vi "Launcher Nested Actor Caller.vi"(8 "error in (no error)":errorcluster, 10 "Sidebar":refnum<vi>, 11 "Post Analysis in":refnum<class "Post Analysis.lvclass">) -> (0 "error out":errorcluster, 3 "Post Analysis out":refnum<class "Post Analysis.lvclass">)   [LabVIEW 2023, in "Data Analysis.lvlib" / "Post Analysis.lvlib" / "Post Analysis.lvclass"]
uses:
  Post Analysis.lvclass
  Post Analysis.lvclass/Post Analysis.ctl
  <vilib>/ActorFramework/Message Enqueuer/Message Enqueuer.lvclass/Message Enqueuer.ctl
  Test Info/Test Info/Test Info.lvclass
  Test Info/Test Info/Test Info.lvclass/Test Info.ctl
  Error Log/Error Log/Error Log.lvclass
  Error Log/Error Log/Error Log.lvclass/Error Log.ctl
  FE FF Frame/FE FF Frame/FE FF Frame.lvclass
  FE FF Frame/FE FF Frame/FE FF Frame.lvclass/FE FF Frame.ctl
  Signal Analysis/Signal Analysis/Signal Analysis.lvclass
  Signal Analysis/Signal Analysis/Signal Analysis.lvclass/Signal Analysis.ctl
  Import Export/Import Export/Export.lvclass
  Import Export/Import Export/Export.lvclass/Export.ctl
  Result Info/Result Info/Result Info.lvclass
  Result Info/Result Info/Result Info.lvclass/Result Info.ctl
  Import Export SQL/Import Export/Import Export SQL.lvclass
  Import Export SQL/Import Export/Import Export SQL.lvclass/Import Export SQL.ctl
  Subpanel-Abstract/Subpanel-Abstract.lvclass/Subpanel-Abstract.ctl
  <vilib>/ActorFramework/Message Enqueuer/Enqueue.vi
  Subpanel-Abstract Messages/Close SP Msg/Close SP Msg.lvclass
  Subpanel-Abstract/Subpanel-Abstract.lvclass
  <vilib>/ActorFramework/Message Priority Queue/Priority Enqueue.vi
  <vilib>/ActorFramework/Message Enqueuer/Message Enqueuer.lvclass
  <vilib>/ActorFramework/Actor/Actor.lvclass
  D:/eDCU LTT/VT LTT Project/Source Code/Data Analysis/Subpanel-Abstract/Subpanel-Abstract.lvclass
  C:/Program Files/National Instruments/LabVIEW 2023/vi.lib/ActorFramework/Actor/Actor.lvclass
  D:/eDCU LTT/VT LTT Project/Source Code/Data Analysis/Test Info/Test Info/Test Info.lvclass
  D:/eDCU LTT/VT LTT Project/Source Code/Data Analysis/Error Log/Error Log/Error Log.lvclass
  D:/eDCU LTT/VT LTT Project/Source Code/Data Analysis/FE FF Frame/FE FF Frame/FE FF Frame.lvclass
  D:/eDCU LTT/VT LTT Project/Source Code/Data Analysis/Signal Analysis/Signal Analysis/Signal Analysis.lvclass
  D:/eDCU LTT/VT LTT Project/Source Code/Data Analysis/Import Export/Import Export/Export.lvclass
  D:/eDCU LTT/VT LTT Project/Source Code/Data Analysis/Result Info/Result Info/Result Info.lvclass
  D:/eDCU LTT/VT LTT Project/Source Code/Data Analysis/Import Export SQL/Import Export/Import Export SQL.lvclass
  D:/eDCU LTT/VT LTT Project/Source Code/Data Analysis/Post Analysis/Post Analysis.lvclass
  Control/SideMenuBar.ctl
  Data Analysis.lvlib
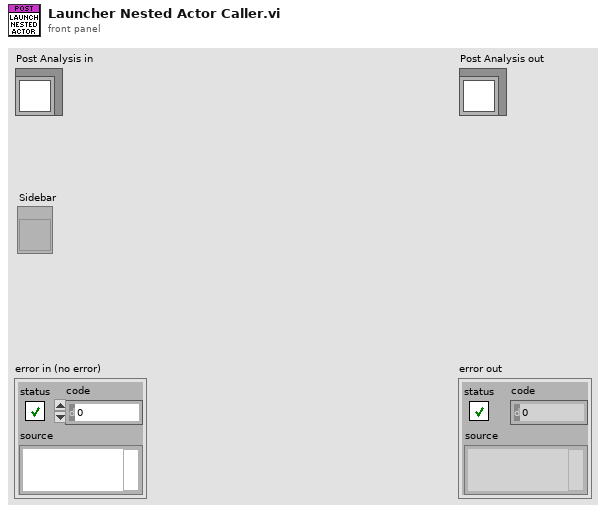
[diagram p1: front panel]
types:
  T1 = typedef "Data Analysis.lvlib/SideMenuBar.ctl" = enum32{"Test Info", "Error Log", "FE/FF Frame", "Signal Analysis", "Export Data", "Test Log Import/Export", "Info"}
  T2 = typedef "Data Analysis.lvlib/Report.ctl" = cluster{"Schema":string, "Test Socket":string, "Start Test Cycle":string, "Stop Test Cycle":string, "Test Mode":string, "Frame Type":string}
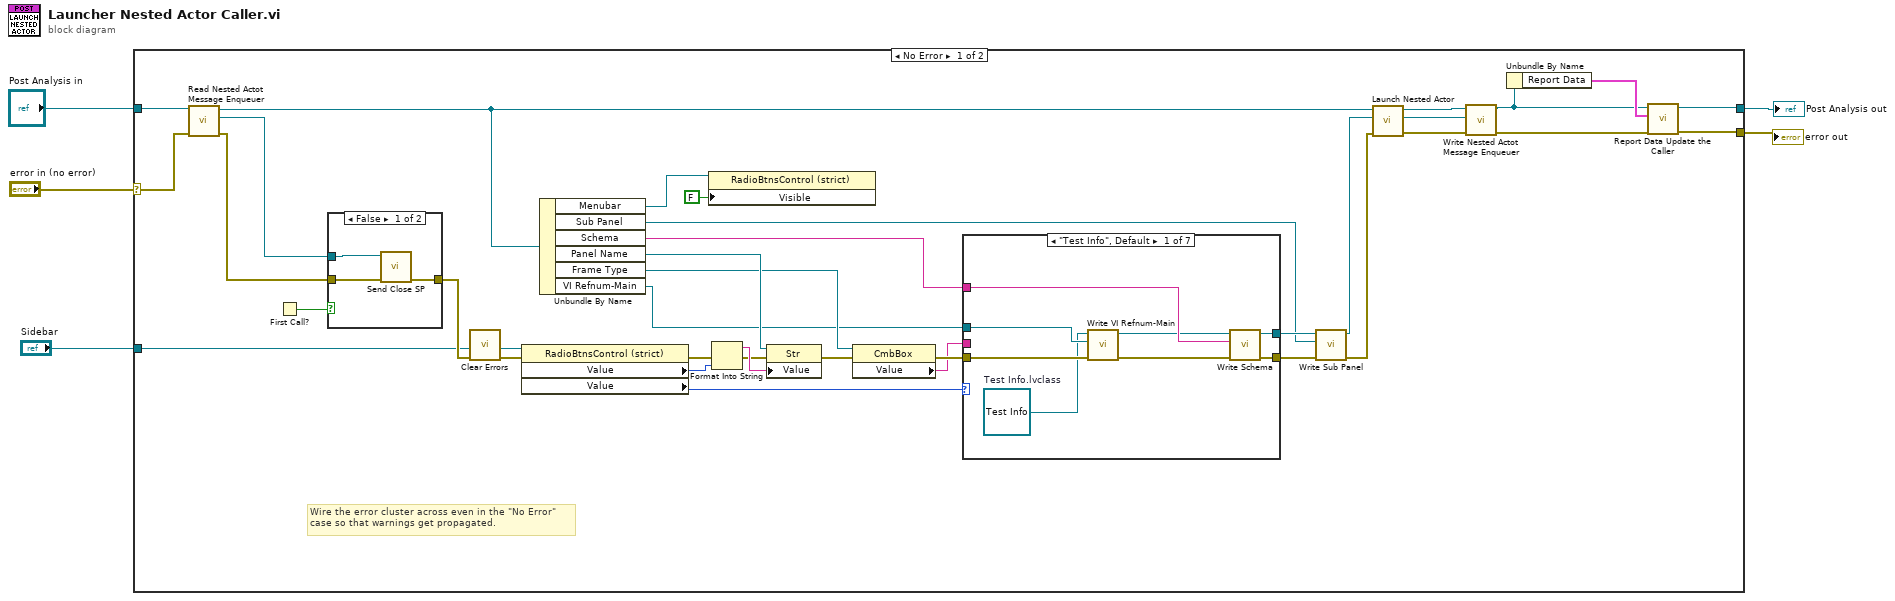
[diagram p0: block diagram]
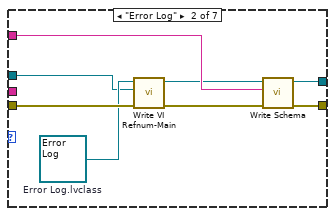
[diagram p2: hidden frame]
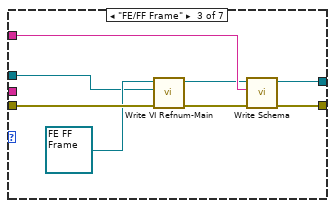
[diagram p3: hidden frame]
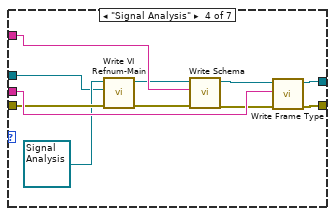
[diagram p4: hidden frame]
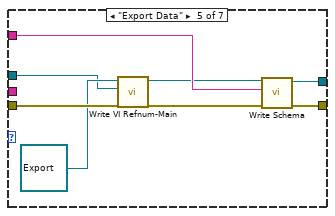
[diagram p5: hidden frame]
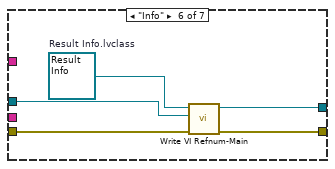
[diagram p6: hidden frame]
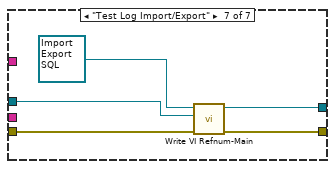
[diagram p7: hidden frame]
diagram:
  n1 = case shown="No Error" "error in (no error)" {
    selector: "error in (no error)" -> [w40 w99]
    tunnel: [w6 w99] -> w4
    tunnel: [w7 w98] -> w2
    tunnel: "Post Analysis in" -> [w41 w98]
    tunnel: "Sidebar" -> [w13 _]
    frame No Error {
      # "Wire the error cluster across even in the \"No Error\"\ncase so that warnings get propagated."
      n2 = call "Read Nested Actot Message Enqueuer.vi"("error in (no error)"=w40, "Post Analysis in"=w41) -> ("error out"=w19:errorcluster, "Actor Framework:Message Enqueuer"=w38:refnum<class "Message Enqueuer.lvclass">, "Post Analysis out"=w10:refnum<class "Post Analysis.lvclass">)  [unwired: 7 in]
      n3 = First Call?() -> (First Call?: T/F=w39:bool)
      n4 = case shown="False" w39 {
        tunnel: w38 -> [w96 _]
        tunnel: [w95 w97] -> w37
        tunnel: w19 -> [w94 w97]
        frame False {
          n5 = call "Send Close SP.vi"("error in (no error)"=w94, "Message Enqueuer"=w96) -> ("error out"=w95:errorcluster)  [unwired: 8 in, 1 out]
        }
        frame True {
        }
      }
      n6 = call <vilib>:"Clear Errors.vi"("error in (no error)"=w37) -> ("error out"=w27:errorcluster)  [unwired: 5 in, 1 out]
      n7 = property class="RadioBtnsControl (strict)"(reference=w13, error in=w27) -> (error out=w22:errorcluster, "Value"=w24:T1, "Value"=w29:T1)  [unwired: 1 out]
      n8 = Unbundle By Name(w10) -> ("Menubar"=w28:refnum<vi>, "Sub Panel"=w35:refnum<vi>, "Schema"=w26:string, "Panel Name"=w25:refnum<vi>, "Frame Type"=w16:refnum<vi>, "VI Refnum-Main"=w14:refnum<vi>)
      n9 = property class="RadioBtnsControl (strict)"(reference=w28, "Visible"=FALSE) -> ()  [unwired: 1 in, 2 out]
      n10 = Format Into String(error in=w22, w24) -> (resulting string=w23:string, error out=w21:errorcluster)  [unwired: 2 in]
      n11 = property class="Str"(reference=w25, error in=w21, "Value"=w23) -> (error out=w18:errorcluster)  [unwired: 1 out]
      n12 = property class="CmbBox"(reference=w16, error in=w18) -> (error out=w17:errorcluster, "Value"=w15:string)  [unwired: 1 out]
      n13 = case shown="\"Test Info\", Default" w29 {
        tunnel: [w49 w57 w65 w74 w83 w85 w93] -> w36
        tunnel: w26 -> [w48 w56 w64 w76 w82 _ _]
        tunnel: w17 -> [w46 w54 w63 w70 w81 w88 w91]
        tunnel: [w47 w55 w59 w71 w80 w87 w90] -> w20
        tunnel: w15 -> [_ _ _ w73 _ _ _]
        tunnel: w14 -> [w43 w50 w58 w66 w77 w84 w89]
        frame "Test Info", Default {
          w42 = refnum<class "Test Info.lvclass"> refnum  # Test Info.lvclass
          n14 = call "Write VI Refnum-Main.vi"("error in (no error)"=w46, "VI Refnum-Main"=w43, "Test Info in"=w42) -> ("error out"=w45:errorcluster, "Test Info out"=w44:refnum<class "Test Info.lvclass">)  [unwired: 7 in]
          n15 = call "Write Schema.vi"("error in (no error)"=w45, "Schema"=w48, "Test Info in"=w44) -> ("error out"=w47:errorcluster, "Test Info out"=w49:refnum<class "Test Info.lvclass">)  [unwired: 7 in]
        }
        frame "Error Log" {
          w52 = refnum<class "Error Log.lvclass"> refnum  # Error Log.lvclass
          n16 = call "Write VI Refnum-Main.vi"("error in (no error)"=w54, "VI Refnum-Main"=w50, "Error Log in"=w52) -> ("error out"=w53:errorcluster, "Error Log out"=w51:refnum<class "Error Log.lvclass">)  [unwired: 7 in]
          n17 = call "Write Schema.vi"("error in (no error)"=w53, "Schema"=w56, "Error Log in"=w51) -> ("error out"=w55:errorcluster, "Error Log out"=w57:refnum<class "Error Log.lvclass">)  [unwired: 7 in]
        }
        frame "FE/FF Frame" {
          n18 = call "Write VI Refnum-Main.vi"("error in (no error)"=w63, "VI Refnum-Main"=w58, "FE FF Frame in"=refnum<class "FE FF Frame.lvclass"> refnum ("Data Analysis.lvlib:FE FF Frame.lvlib:FE FF Frame.lvclass")) -> ("error out"=w60:errorcluster, "FE FF Frame out"=w61:refnum<class "FE FF Frame.lvclass">)  [unwired: 7 in]
          n19 = call "Write Schema.vi"("error in (no error)"=w60, "Schema"=w64, "FE FF Frame in"=w61) -> ("error out"=w59:errorcluster, "FE FF Frame out"=w65:refnum<class "FE FF Frame.lvclass">)  [unwired: 7 in]
        }
        frame "Signal Analysis" {
          n20 = call "Write VI Refnum-Main.vi"("error in (no error)"=w70, "VI Refnum-Main"=w66, "Signal Analysis in"=refnum<class "Signal Analysis.lvclass"> refnum ("Data Analysis.lvlib:Signal Analysis.lvlib:Signal Analysis.lvclass")) -> ("error out"=w69:errorcluster, "Signal Analysis out"=w67:refnum<class "Signal Analysis.lvclass">)  [unwired: 7 in]
          n21 = call "Write Schema.vi"("error in (no error)"=w69, "Schema"=w76, "Signal Analysis in"=w67) -> ("error out"=w72:errorcluster, "Signal Analysis out"=w75:refnum<class "Signal Analysis.lvclass">)  [unwired: 7 in]
          n22 = call "Write Frame Type.vi"("error in (no error)"=w72, "Frame Type"=w73, "Signal Analysis in"=w75) -> ("error out"=w71:errorcluster, "Signal Analysis out"=w74:refnum<class "Signal Analysis.lvclass">)  [unwired: 7 in]
        }
        frame "Export Data" {
          n23 = call "Write VI Refnum-Main.vi"("VI Refnum-Main"=w77, "Import Export in"=refnum<class "Export.lvclass"> refnum ("Data Analysis.lvlib:Import Export.lvlib:Import Export.lvclass")) -> ("Import Export out"=w78:refnum<class "Export.lvclass">)  [unwired: 8 in, 1 out]
          n24 = call "Write Schema.vi"("error in (no error)"=w81, "Schema"=w82, "Import Export in"=w78) -> ("error out"=w80:errorcluster, "Import Export out"=w83:refnum<class "Export.lvclass">)  [unwired: 7 in]
        }
        frame "Info" {
          w86 = refnum<class "Result Info.lvclass"> refnum  # Result Info.lvclass
          n25 = call "Write VI Refnum-Main.vi"("error in (no error)"=w88, "VI Refnum-Main"=w84, "Result Info in"=w86) -> ("error out"=w87:errorcluster, "Result Info out"=w85:refnum<class "Result Info.lvclass">)  [unwired: 7 in]
        }
        frame "Test Log Import/Export" {
          n26 = call "Write VI Refnum-Main.vi"("error in (no error)"=w91, "VI Refnum-Main"=w89, "Import Export in"=refnum<class "Import Export SQL.lvclass"> refnum ("Data Analysis.lvlib:Import Export SQL.lvlib:Import Export SQL.lvclass")) -> ("error out"=w90:errorcluster, "Import Export out"=w93:refnum<class "Import Export SQL.lvclass">)  [unwired: 7 in]
        }
      }
      n27 = call "Write Sub Panel.vi"("error in (no error)"=w20, "Sub Panel"=w35, "Subpanel-Abstract in"=w36) -> ("error out"=w11:errorcluster, "Subpanel-Abstract out"=w34:refnum<class "Subpanel-Abstract.lvclass">)  [unwired: 7 in]
      n28 = call <vilib>:"Launch Nested Actor.vi"("error in (no error)"=w11, "Nested Actor"=w34, "Caller Actor in"=w10) -> ("error out"=w32:errorcluster, "Nested Actor's Enqueuer"=w31:refnum<class "Message Enqueuer.lvclass">, "Caller Actor out"=w33:refnum<class "Post Analysis.lvclass">)  [unwired: 6 in]
      n29 = call "Write Nested Actot Message Enqueuer.vi"("error in (no error)"=w32, "Actor Framework:Message Enqueuer"=w31, "Post Analysis in"=w33) -> ("error out"=w8:errorcluster, "Post Analysis out"=w9:refnum<class "Post Analysis.lvclass">)  [unwired: 7 in]
      n30 = Unbundle By Name(w9) -> ("Report Data"=w12:T2)
      n31 = call "Report Data Update the Caller.vi"("error in (no error)"=w8, "Report Data"=w12, "Post Analysis in"=w9) -> ("error out"=w6:errorcluster, "Post Analysis out"=w7:refnum<class "Post Analysis.lvclass">)  [unwired: 7 in]
    }
    frame Error {
    }
  }
  "error out" <- w4
  "Post Analysis out" <- w2
